vi "ConfigurationDatabase_Module.vi"(8 "error in":errorcluster) -> (0 "error out":errorcluster, 3 "Data_Dummy":T1)   [LabVIEW 2019]
uses:
  #typedef_Data_Cluster.ctl
  #typedef_EntryConsole_Action_enum.ctl
  #typedef_WashDisplay_Action_enum.ctl
  #typedef_Controller_Action_enum.ctl
  #typedef_VehiclePosition_Action_enum.ctl
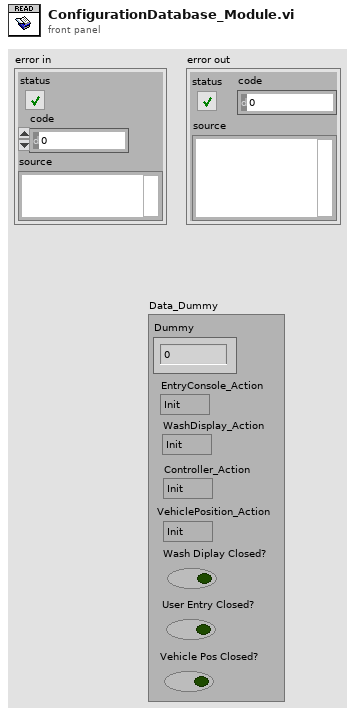
[diagram p1: front panel]
types:
  T1 = typedef "#typedef_Data_Cluster.ctl" = cluster{"Dummy":dbl, "EntryConsole_Action":T2, "WashDisplay_Action":T3, "Controller_Action":T4, "VehiclePosition_Action":T5, "Wash Diplay Closed?":bool, "User Entry Closed?":bool, "Vehicle Pos Closed? ":bool}
  T2 = typedef "#typedef_EntryConsole_Action_enum.ctl" = enum16{"Init", "ERROR_DEFAULT", "Idle", "Specific", "Close", "Error_Handler", "Exit"}
  T3 = typedef "#typedef_WashDisplay_Action_enum.ctl" = enum16{"Init", "ERROR_DEFAULT", "Idle", "Specific", "Close", "Error_Handler", "Exit"}
  T4 = typedef "#typedef_Controller_Action_enum.ctl" = enum16{"Init", "ERROR_DEFAULT", "Idle", "Read database", "Close", "Error_Handler", "Exit"}
  T5 = typedef "#typedef_VehiclePosition_Action_enum.ctl" = enum16{"Init", "ERROR_DEFAULT", "Idle", "Specific", "Close", "Error_Handler", "Exit"}
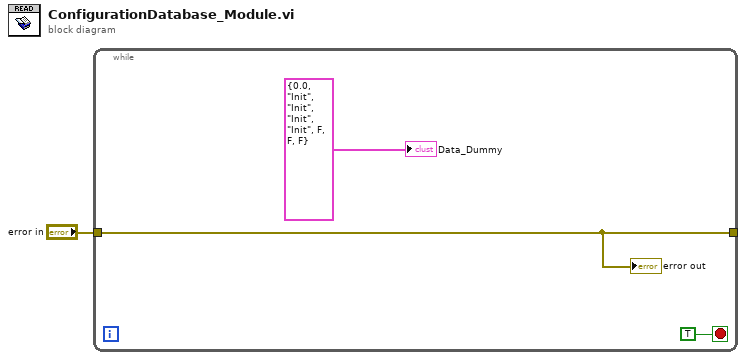
[diagram p0: block diagram]
diagram:
  n1 = while {
    tunnel: "error in" -> [w2]
    tunnel: [w2] -> _
    stop <- TRUE stop-if-true
    "Data_Dummy" <- T1 {"Dummy"=0.0, "EntryConsole_Action"=enum."Init", "WashDisplay_Action"=enum."Init", "Controller_Action"=enum."Init", "VehiclePosition_Action"=enum."Init", "Wash Diplay Closed?"=FALSE, "User Entry Closed?"=FALSE, "Vehicle Pos Closed? "=FALSE} ("Data_VehiclePos")
    "error out" <- w2
  }
